vi "SeCrTs-Event Handler.vi"(8 "error in (no error)":errorcluster, 10 "Ev":refnum<queue>, 11 "CtlRef":refnum<vi>) -> (0 "error out":errorcluster)   [LabVIEW 2022 SP3]
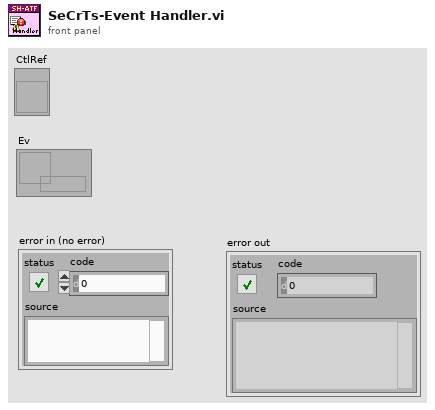
[diagram p1: front panel]
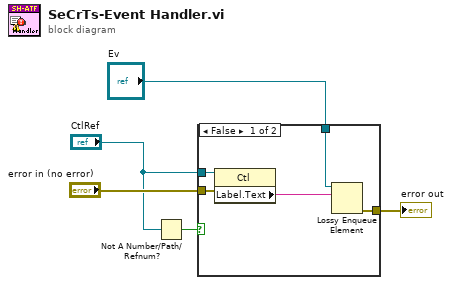
[diagram p0: block diagram]
diagram:
  n1 = Not A Number/Path/Refnum?(number/path/refnum="CtlRef") -> (NaN/Path/Refnum?=w2:bool)
  n2 = case shown="False" w2 {
    tunnel: "CtlRef" -> [w10 _]
    tunnel: "Ev" -> [w8 _]
    tunnel: [w7 w11] -> w4
    tunnel: "error in (no error)" -> [w6 w11]
    frame False {
      n3 = property class="Ctl"(reference=w10, error in=w6) -> ("Label.Text"=w9:string)  [unwired: 2 out]
      n4 = Lossy Enqueue Element(queue=w8, element=w9) -> (error out=w7:errorcluster)  [unwired: 1 in, 3 out]
    }
    frame True {
    }
  }
  "error out" <- w4
